vi "Connect.vi"(4 "timeout (5000 ms)":u32=5000, 7 "username/password":cluster{"username":string, "password":string}, 8 "error in (no error)":errorcluster, 9 "client certificate file":path, 10 "Server IP":string, 11 "XML config File Path":path=path "D:/work/Project support in lanzhou/OPCUA XML/xml/server config.xml") -> (0 "error out":errorcluster, 1 "OPC UA data change event":refnum<user-event>, 2 "server endpoint URL":string, 3 "OPC UA client refnum out":refnum<k21>, 5 "trusted Server certfications":path[](array[path]))   [LabVIEW 2013, in "OCPUA Client(UtilityMode).lvlib"]
uses:
  OCPUA Client(UtilityMode).lvlib
  _op(client).ctl
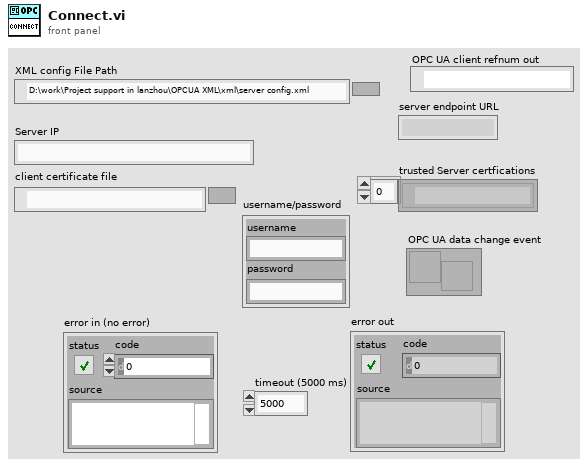
[diagram p1: front panel]
types:
  T1 = typedef "OCPUA Client(UtilityMode).lvlib/_op(client).ctl" = enum16{"Connect Server", "Get Client Refnum", "Disconnect Server"}
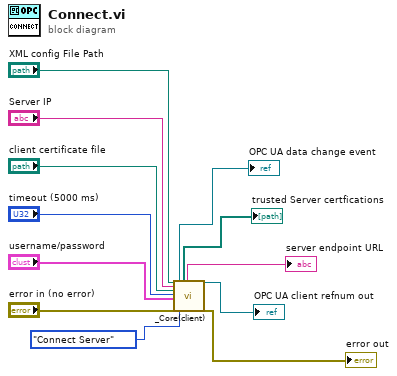
[diagram p0: block diagram]
diagram:
  n1 = call "_Core(client).vi"("XML config File Path"="XML config File Path", "Server IP"="Server IP", "client cert path(empty path)"="client certificate file", "timeout (5000 ms)"="timeout (5000 ms)", "username/password"="username/password", "error in (no error)"="error in (no error)", "Op"=_op(client)."Connect Server") -> ("OPC UA data change event"=→"OPC UA data change event":refnum<user-event>, "trusted Server certfications"=→"trusted Server certfications":path[], "server endpoint URL"=→"server endpoint URL":string, "OPC UA client refnum out"=→"OPC UA client refnum out":refnum<k21>, "error out"=→"error out":errorcluster)  [unwired: 16 in]
